vi "Create Label or Caption Object.vi"(6 "Cluster Component":bool, 7 "Text Type":T1, 8 "error in (no error)":errorcluster, 10 "GObject":refnum<vi>, 11 "Text in":refnum<class "Text.lvclass">) -> (0 "error out":errorcluster, 3 "Text out":refnum<class "Text.lvclass">)   [LabVIEW 2017, in "Front Panel Publisher.lvlib" / "Text.lvclass"]
uses:
  Text.lvclass
  Enum - Create Text Method.ctl
  Object_class/Coordinates.ctl
  Object_class/Attributes.ctl
  <vilib>/Utility/miscctls.llb/LVRectTypeDef.ctl
  Object_class/Enum - Pane Coordinate Method.ctl
  Text.lvclass/Text.ctl
  Object_class/Object.lvclass
  Front Panel Publisher.lvlib
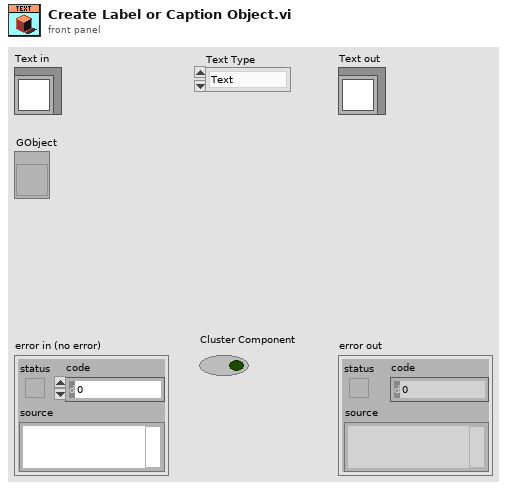
[diagram p1: front panel]
types:
  T1 = typedef "Front Panel Publisher.lvlib/Text.lvclass/Enum - Create Text Method.ctl" = enum16{"Text", "Label", "Caption", "Boolean Text"}
  T2 = typedef "Front Panel Publisher.lvlib/Object.lvclass/Coordinates.ctl" = cluster{"Left":i32, "Top":i32, "Height":u32, "Width":u32}
  T3 = typedef "Front Panel Publisher.lvlib/Object.lvclass/Enum - Pane Coordinate Method.ctl" = enum16{"Initialize", "Get Last Pane Offset", "Update Pane Position"}
  T4 = typedef "Front Panel Publisher.lvlib/Object.lvclass/Attributes.ctl" = cluster{"UID":i32, "Type":string, "Starting Location":T2, "Reference":refnum<vi>, "Cluster Component":bool, "Starting Rect Position":cluster{"Left":i16, "Top":i16}, "Owning Pane":refnum<vi>, "Master Total Rect Delta":T5}
  T5 = typedef "LVRectTypeDef.ctl" = cluster{"Left":i16, "Top":i16, "Right":i16, "Bottom":i16}
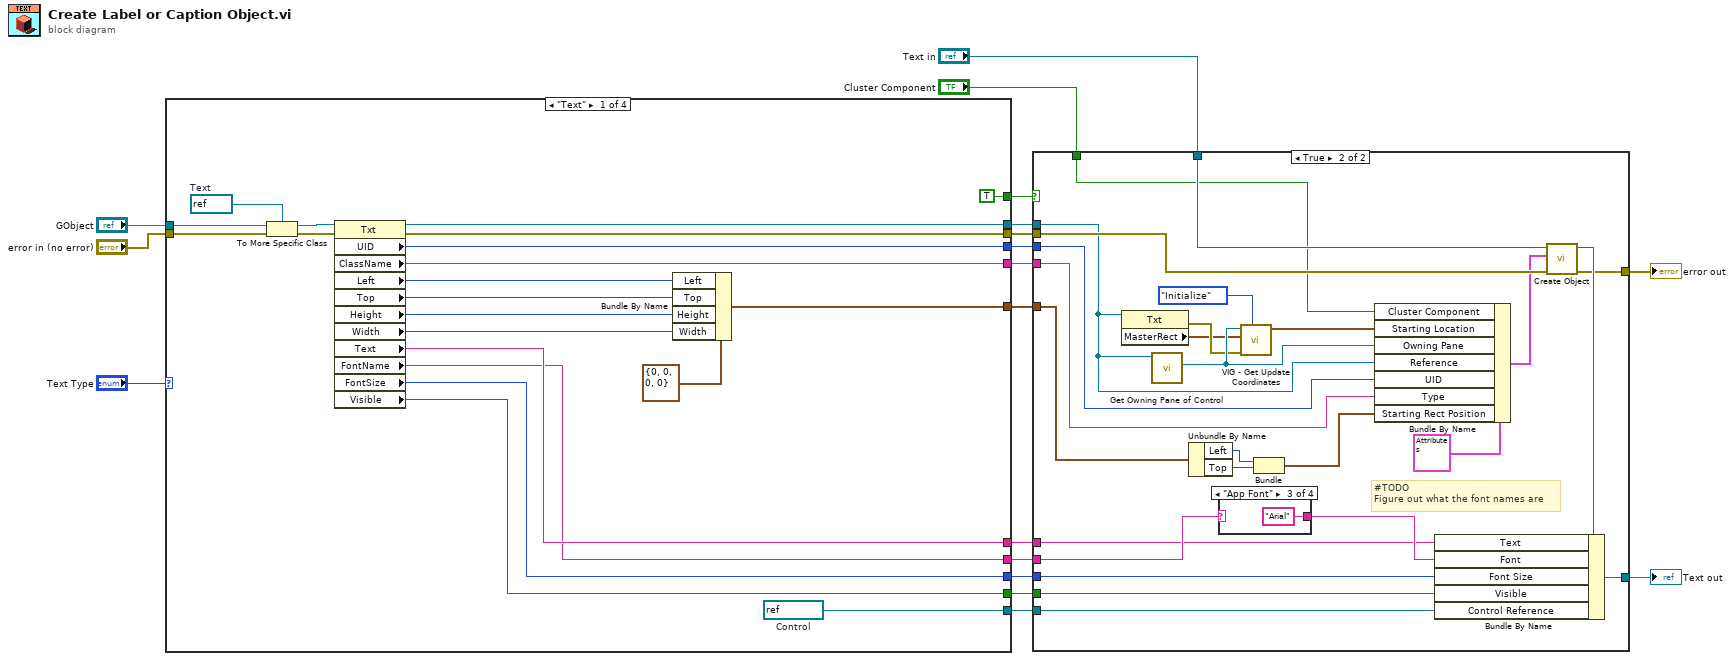
[diagram p0: block diagram]
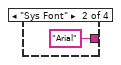
[diagram p4: hidden frame]
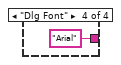
[diagram p5: hidden frame]
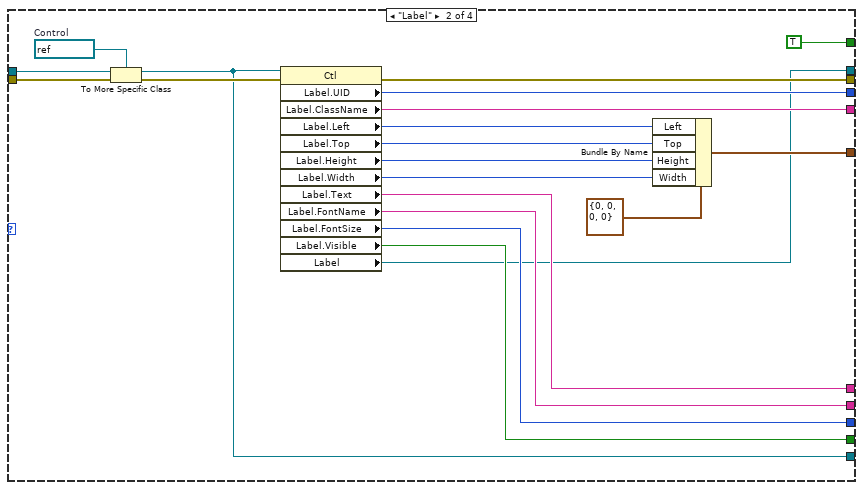
[diagram p6: hidden frame]
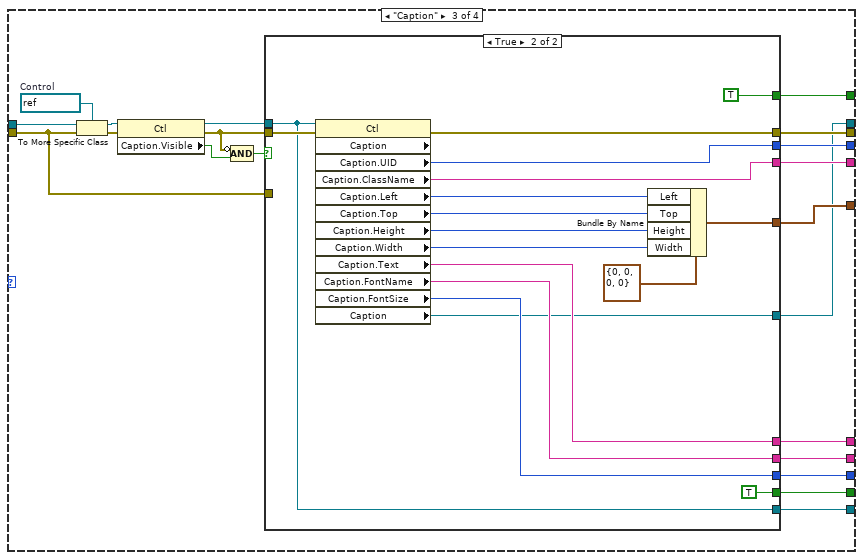
[diagram p7: hidden frame]
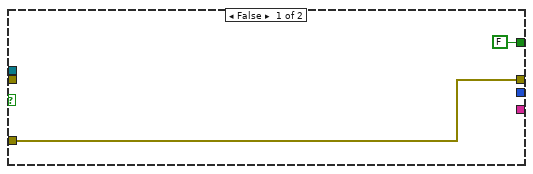
[diagram p8: hidden frame]
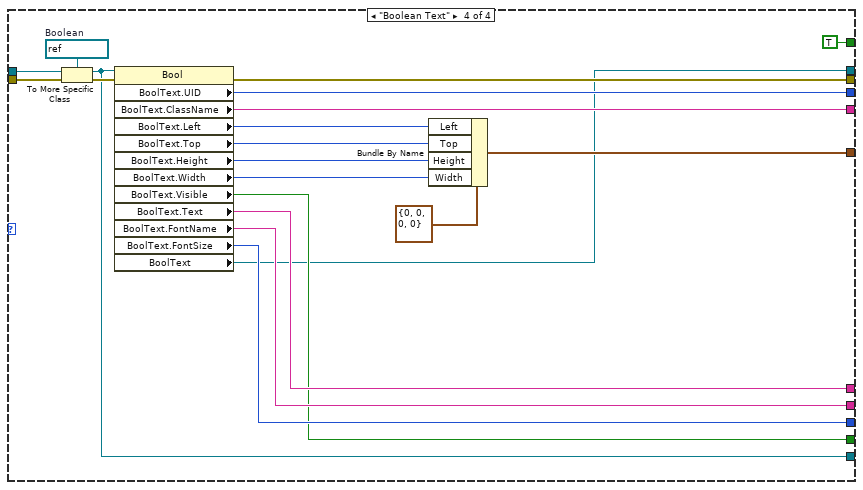
[diagram p9: hidden frame]
diagram:
  n1 = case shown="\"Text\"" "Text Type" {
    tunnel: "GObject" -> [w32 w53 w72 w112]
    tunnel: [w28 w52 w70 w105] -> w15
    tunnel: [w29 w51 w69 w104] -> w14
    tunnel: [w30 w50 w68 w108] -> w13
    tunnel: [w20 w49 w63 w107] -> w12
    tunnel: [w21 w48 w62 w106] -> w11
    tunnel: [w25 w47 w67 w101] -> w9
    tunnel: [w24 w46 w66 w102] -> w8
    tunnel: [w26 w44 w65 w103] -> w7
    tunnel: "error in (no error)" -> [w31 w43 w71 w111]
    tunnel: [w23 w42 w64 w110] -> w5
    tunnel: [TRUE TRUE w61 TRUE] -> w3
    tunnel: [w19 w40 w60 w99] -> w2
    frame "Text" {
      w28 = refnum<vi> refnum  # Control
      w38 = refnum<vi> refnum  # Text
      n2 = To More Specific Class(target class=w38, reference=w32, error in=w31) -> (specific class reference=w33:refnum<vi>, error out=w39:errorcluster)
      n3 = property class="Txt"(reference=w33, error in=w39) -> (reference out=w19:refnum<vi>, error out=w23:errorcluster, "UID"=w25:i32, "ClassName"=w24:string, "Left"=w37:i32, "Top"=w36:i32, "Height"=w35:u32, "Width"=w34:u32, "Text"=w21:string, "FontName"=w20:string, "FontSize"=w30:u32, "Visible"=w29:bool)
      n4 = Bundle By Name(cluster=T2 {"Left"=0, "Top"=0, "Height"=0, "Width"=0} ("Coordinates"), "Left"=w37, "Top"=w36, "Height"=w35, "Width"=w34) -> (w26:T2)
    }
    frame "Label" {
      w58 = refnum<vi> refnum  # Control
      n5 = To More Specific Class(target class=w58, reference=w53, error in=w43) -> (specific class reference=w52:refnum<vi>, error out=w59:errorcluster)
      n6 = property class="Ctl"(reference=w52, error in=w59) -> (error out=w42:errorcluster, "Label.UID"=w47:i32, "Label.ClassName"=w46:string, "Label.Left"=w57:i32, "Label.Top"=w56:i32, "Label.Height"=w55:u32, "Label.Width"=w54:u32, "Label.Text"=w48:string, "Label.FontName"=w49:string, "Label.FontSize"=w50:u32, "Label.Visible"=w51:bool, "Label"=w40:refnum<vi>)  [unwired: 1 out]
      n7 = Bundle By Name(cluster=T2 {"Left"=0, "Top"=0, "Height"=0, "Width"=0} ("Coordinates"), "Left"=w57, "Top"=w56, "Height"=w55, "Width"=w54) -> (w44:T2)
    }
    frame "Caption" {
      w77 = refnum<vi> refnum  # Control
      n8 = To More Specific Class(target class=w77, reference=w72, error in=w71) -> (specific class reference=w76:refnum<vi>, error out=w79:errorcluster)
      n9 = property class="Ctl"(reference=w76, error in=w79) -> (reference out=w73:refnum<vi>, error out=w78:errorcluster, "Caption.Visible"=w75:bool)
      n10 = Compound Arithmetic op=AND(invert w78, w75) -> (w74:bool)
      n11 = case shown="True" w74 {
        tunnel: w73 -> [_ w92]
        tunnel: w78 -> [_ w98]
        tunnel: [w81 w86] -> w64
        tunnel: w71 -> [w81 _]
        tunnel: [_ w92] -> w70
        tunnel: [_ TRUE ("Visible")] -> w69
        tunnel: [_ w90] -> w68
        tunnel: [_ w89] -> w67
        tunnel: [_ w88] -> w66
        tunnel: [_ w87] -> w65
        tunnel: [_ w85] -> w63
        tunnel: [_ w84] -> w62
        tunnel: [FALSE TRUE] -> w61
        tunnel: [_ w82] -> w60
        frame False {
        }
        frame True {
          n12 = property class="Ctl" props=["Caption", "Caption", "UID", "Caption", "ClassName", "Caption", "Left", "Caption", "Top", "Caption", "Height", "Caption", "Width", "Caption", "Text", "Caption", "FontName", "Caption", "FontSize", "Caption"](reference=w92, error in=w98) -> (error out=w86:errorcluster, "Caption.UID"=w89:i32, "Caption.ClassName"=w88:string, "Caption.Left"=w97:i32, "Caption.Top"=w96:i32, "Caption.Height"=w95:u32, "Caption.Width"=w94:u32, "Caption.Text"=w84:string, "Caption.FontName"=w85:string, "Caption.FontSize"=w90:u32, "Caption"=w82:refnum<vi>)  [unwired: 2 out]
          n13 = Bundle By Name(cluster=T2 {"Left"=0, "Top"=0, "Height"=0, "Width"=0} ("Coordinates"), "Left"=w97, "Top"=w96, "Height"=w95, "Width"=w94) -> (w87:T2)
        }
      }
    }
    frame "Boolean Text" {
      w118 = refnum<vi> refnum  # Boolean
      n14 = To More Specific Class(target class=w118, reference=w112, error in=w111) -> (specific class reference=w105:refnum<vi>, error out=w113:errorcluster)
      n15 = property class="Bool"(reference=w105, error in=w113) -> (error out=w110:errorcluster, "BoolText.UID"=w101:i32, "BoolText.ClassName"=w102:string, "BoolText.Left"=w117:i32, "BoolText.Top"=w116:i32, "BoolText.Height"=w115:u32, "BoolText.Width"=w114:u32, "BoolText.Visible"=w104:bool, "BoolText.Text"=w106:string, "BoolText.FontName"=w107:string, "BoolText.FontSize"=w108:u32, "BoolText"=w99:refnum<vi>)  [unwired: 1 out]
      n16 = Bundle By Name(cluster=T2 {"Left"=0, "Top"=0, "Height"=0, "Width"=0} ("Coordinates"), "Left"=w117, "Top"=w116, "Height"=w115, "Width"=w114) -> (w103:T2)
    }
  }
  n17 = case shown="True" w3 {
    tunnel: [w119 w145] -> w18
    tunnel: "Text in" -> [w119 w144]
    tunnel: w15 -> [_ w142]
    tunnel: w14 -> [_ w141]
    tunnel: w13 -> [_ w140]
    tunnel: w12 -> [_ w139]
    tunnel: w11 -> [_ w138]
    tunnel: w9 -> [_ w131]
    tunnel: w8 -> [_ w130]
    tunnel: w7 -> [_ w127]
    tunnel: w5 -> [w120 w137]
    tunnel: [w120 w136] -> w4
    tunnel: w2 -> [_ w122]
    tunnel: "Cluster Component" -> [_ w132]
    frame False {
    }
    frame True {
      # "#TODO\nFigure out what the font names are"
      n18 = property class="Txt"(reference=w122) -> (error out=w124:errorcluster, "MasterRect"=w123:T5)  [unwired: 1 in, 1 out]
      n19 = call "Get Owning Pane of Control.vi"("GObj Refnum"=w122) -> ("Owning Pane"=w135:refnum<vi>)  [unwired: 7 in, 3 out]
      n20 = Unbundle By Name(w127) -> ("Left"=w128:i32, "Top"=w129:i32)
      n21 = case shown="\"App Font\"" w139 {
        selector: w139 -> [w147 _ _ _]
        tunnel: [w147 "Arial" "Arial" "Arial"] -> w146
        frame Default {
        }
        frame "Sys Font" {
        }
        frame "App Font" {
        }
        frame "Dlg Font" {
        }
      }
      n22 = call "VIG - Get Update Coordinates.vi"("Pane Method"=Enum_-_Pane_Coordinate_Method."Initialize", "error in (no error)"=w124, "MasterRect"=w123, "Pane in"=w135) -> ("Coordinates"=w134:T2)  [unwired: 5 in, 2 out]
      n23 = Bundle("Left"=w128, "Top"=w129) -> (w126:cluster{"Left":i32, "Top":i32})  [unwired: 1 in]
      n24 = Bundle By Name(cluster=T4 {"UID"=0, "Type"="", "Starting Location"={"Left"=0, "Top"=0, "Height"=0, "Width"=0}, "Reference"=refnum, "Cluster Component"=FALSE, "Starting Rect Position"={"Left"=0, "Top"=0}, "Owning Pane"=refnum, "Master Total Rect Delta"={"Left"=0, "Top"=0, "Right"=0, "Bottom"=0}} ("Object Attributes"), "Cluster Component"=w132, "Starting Location"=w134, "Owning Pane"=w135, "Reference"=w122, "UID"=w131, "Type"=w130, "Starting Rect Position"=w126) -> (w125:T4)
      n25 = call-dynamic "Create Object.vi"("error in (no error)"=w137, "Object Attributes"=w125, "GObject in"=w144) -> ("error out"=w136:errorcluster, "GObject out"=w143:refnum<class "Text.lvclass">)  [unwired: 7 in]
      n26 = Bundle By Name(cluster=w143, "Text"=w138, "Font"=w146, "Font Size"=w140, "Visible"=w141, "Control Reference"=w142) -> (w145:refnum<class "Text.lvclass">)
    }
  }
  "Text out" <- w18
  "error out" <- w4
